vi "Drive Train.vi"(0 "C":dbl format="%#_13g", 1 "D":dbl format="%#_13g", 2 "X":dbl format="%#_13g", 3 "Y":dbl format="%#_13g", 4 "gyro":dbl, 6 "Mode Switch":bool, 7 "Button 2":bool=TRUE, 8 "Button 1":bool, 9 "Button 3":bool) -> (12 "gyro angle":dbl, 14 "A":dbl, 15 "B":dbl, 16 "R":dbl format="%#_13g")   [LabVIEW 2014]
panel:
  in  "Turning Switch":bool
  in  "alpha":dbl
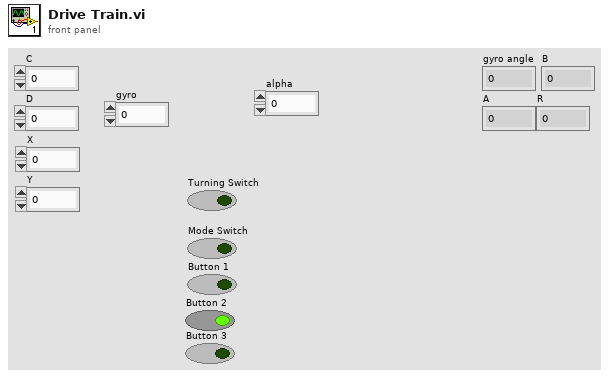
[diagram p1: front panel]
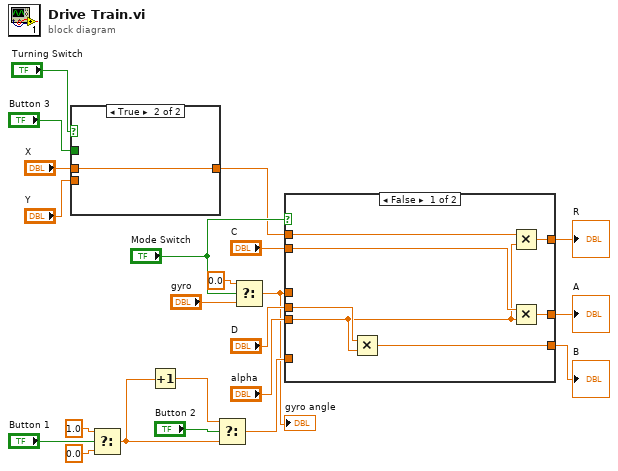
[diagram p0: block diagram]
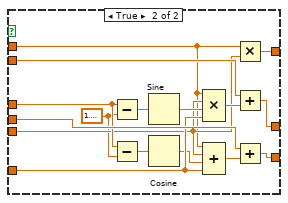
[diagram p2: hidden frame]
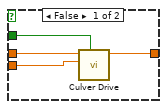
[diagram p3: hidden frame]
diagram:
  n1 = case shown="True" "Turning Switch" {
    tunnel: [w24 w27] -> w10
    tunnel: "X" -> [w25 w27]
    tunnel: "Y" -> [w26 _]
    tunnel: "Button 3" -> [w23 _]
    frame False {
      n2 = call "Culver Drive.vi"("X"=w25, "Y"=w26, "Toggle R"=w23) -> ("R"=w24:ext)  [unwired: 7 in]
    }
    frame True {
    }
  }
  n3 = Select(t=1.0, s="Button 1", f=0.0) -> (s? t:f=w17:dbl)
  n4 = Increment(x=w17) -> (x+1=w16:dbl)
  n5 = Select(t=w16, s="Button 2", f=w17) -> (s? t:f=w11:dbl)
  n6 = Select(t=0.0, s="Mode Switch", f="gyro") -> (s? t:f=w7:dbl)
  "gyro angle" <- w7
  n7 = case shown="False" "Mode Switch" {
    tunnel: "C" -> [w31 w49]
    tunnel: "D" -> [w34 w47]
    tunnel: w10 -> [w30 w36]
    tunnel: w11 -> [_ w46]
    tunnel: "alpha" -> [w28 w37]
    tunnel: w7 -> [_ w41]
    tunnel: [w32 w40] -> w6
    tunnel: [w33 w39] -> w5
    tunnel: [w29 w38] -> w4
    frame False {
      n8 = Multiply(x=w34, y=w28) -> (x*y=w33:dbl)
      n9 = Multiply(x=w30, y=w28) -> (x*y=w29:ext)
      n10 = Multiply(x=w31, y=w28) -> (x*y=w32:dbl)
    }
    frame True {
      w35 = 1.5707963267948966
      n11 = Subtract(x=w41, y=w35) -> (x-y=w43:dbl)
      n12 = Subtract(x=w41, y=w35) -> (x-y=w42:dbl)
      n13 = Sine(x=w43) -> (sin(x)=w45:dbl)
      n14 = Cosine(x=w42) -> (cos(x)=w44:dbl)
      n15 = Compound Arithmetic op=MULTIPLY(w36, w37, w45, w46) -> (w48:ext)
      n16 = Compound Arithmetic op=ADD(w36, w37, w44, w46) -> (w50:ext)
      n17 = Multiply(x=w36, y=w37) -> (x*y=w38:ext)
      n18 = Add(x=w49, y=w48) -> (x+y=w40:ext)
      n19 = Add(x=w47, y=w50) -> (x+y=w39:ext)
    }
  }
  "A" <- w6
  "B" <- w5
  "R" <- w4
